vi "OOB Checker.vi"(8 "Deform Array":dbl[](array[numeric])=[1.0, 1.0, 1.0, 0.0, 0.0, 0.0, 0.0, 0.0, 0.0], 9 "Eye Model Cluster":T2={"X Grid"=[], "Y Grid"=[], "Za_true Surf"=[], "Iris Center"=[], "Zp_true Surf"=[], "Pinv"=[[1.0, 0.0], [0.0, 1.0]], "za_true"=5.0, "za_work"=1.0, "zp_work"=-1.0, "zp_true"=-5.0}, 11 "Check Pt":dbl[](array[numeric])=[0.0, 0.0, 0.0]) -> (0 "Point Out of Bound":bool, 3 "Check Pt*":dbl[](array[numeric]))   [LabVIEW 2016]
uses:
  <vilib>/Analysis/Matrix/Datatypes/RealMatrix.ctl
  <vilib>/Analysis/baseanly.llb/A x Vector.vi
  Subsystems/Global Variables.vi
  <vilib>/Analysis/baseanly.llb/Real Inverse Matrix.vi
  <vilib>/Analysis/7linalg.llb/Create Special Real Matrix.vi
  <vilib>/Analysis/NI_AALBase.lvlib
  <vilib>/Analysis/NI_AALPro.lvlib
  <vilib>/Analysis/NI_AALBLAS.lvlib
  <vilib>/Analysis/Matrix/NI_Matrix.lvlib
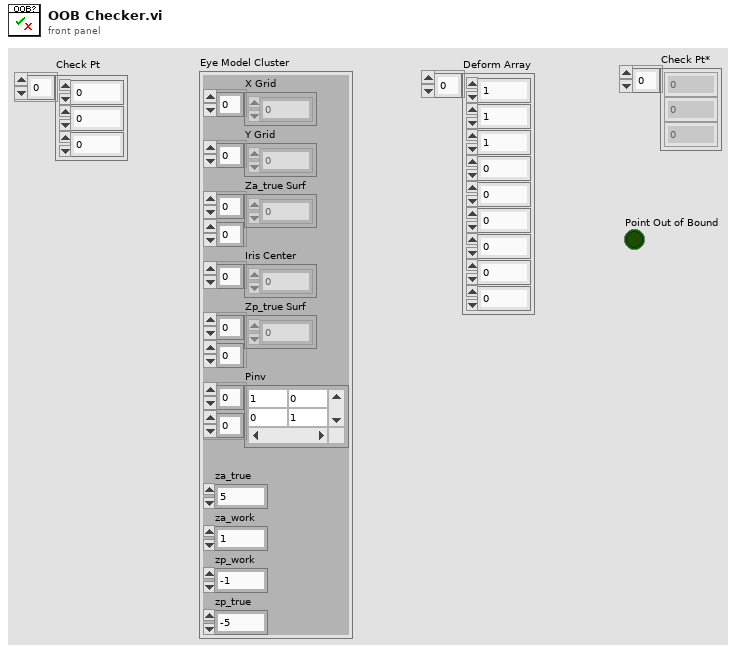
[diagram p1: front panel]
types:
  T1 = typedef "NI_Matrix.lvlib/RealMatrix.ctl" = dbl[][]
  T2 = cluster{"X Grid":dbl[], "Y Grid":dbl[], "Za_true Surf":dbl[][], "Iris Center":dbl[], "Zp_true Surf":dbl[][], "Pinv":T1, "za_true":dbl, "za_work":dbl, "zp_work":dbl, "zp_true":dbl}
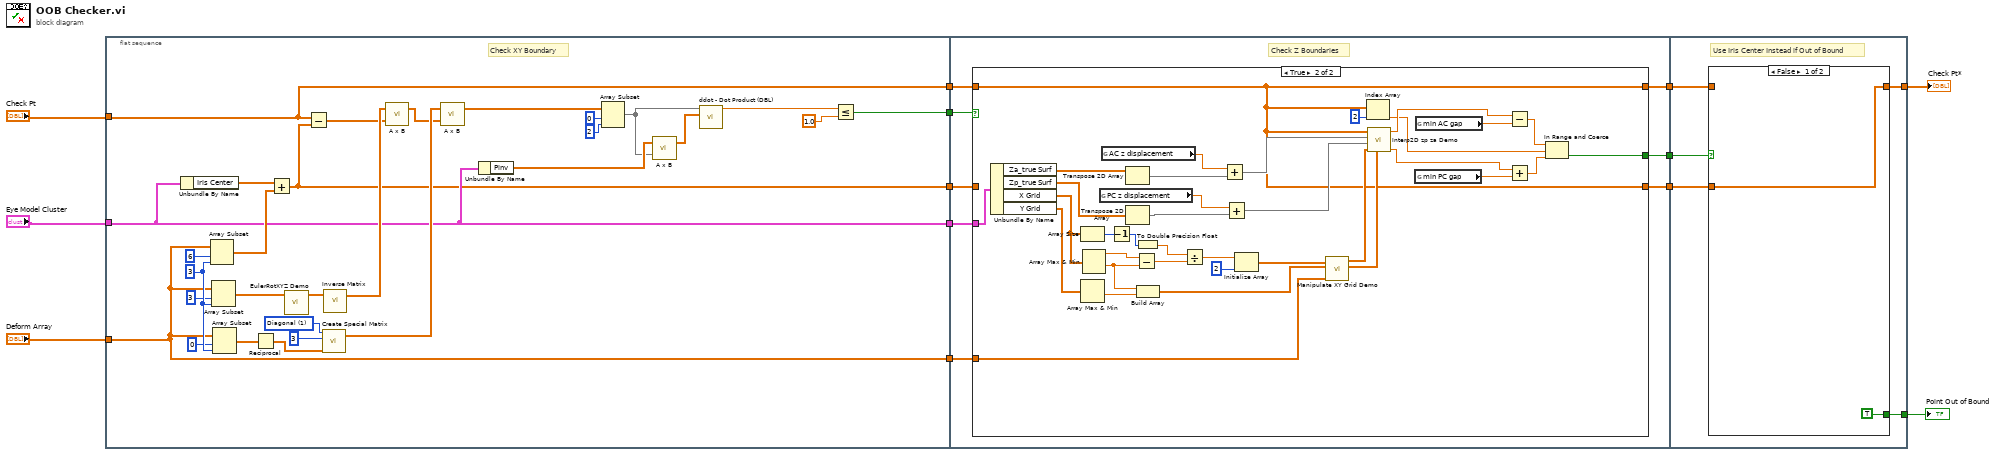
[diagram p0: block diagram]
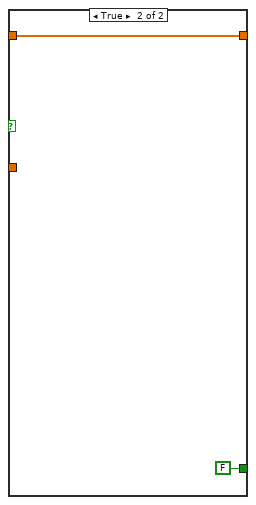
[diagram p3: hidden frame]
diagram:
  n1 = flat-sequence {
    tunnel: [w23] -> w13
    tunnel: [w15] -> w12
    tunnel: [w16] -> w11
    tunnel: [w17] -> w10
    tunnel: "Deform Array" -> [w17]
    tunnel: "Check Pt" -> [w15]
    tunnel: "Eye Model Cluster" -> [w16]
    tunnel: [w14] -> w4
    tunnel: w13 -> [w50]
    tunnel: w12 -> [w48]
    tunnel: w11 -> [w49]
    tunnel: w10 -> [w47]
    tunnel: [w46] -> w9
    tunnel: [w45] -> w8
    tunnel: w4 -> [w44]
    tunnel: [w43] -> w2
    tunnel: w9 -> [w93]
    tunnel: [w92] -> w3
    tunnel: w8 -> [w90]
    tunnel: [w91] -> w1
    tunnel: w2 -> [w89]
    frame #0 {
      w31 = 1 items=["Identity", "Diagonal", "Toeplitz", "Vandermonde", "Companion", "Hankel", "Hadamard", "Wilkinson", "Hilbert", "Inverse Hilbert", "Rosser", "Pascal"] ("matrix type")
      w41 = 3 ("length")
      # "Check XY Boundary"
      n2 = Unbundle By Name(w16) -> ("Iris Center"=w28:dbl[])
      n3 = Array Subset(array=w17, index=6 ("length"), length=w41) -> (w27:dbl[])
      n4 = Array Subset(array=w17, index=3, length=w41) -> (w38:dbl[])
      n5 = Array Subset(array=w17, index=0, length=w41) -> (w34:dbl[])
      n6 = Reciprocal(x=w34) -> (1/x=w33:dbl[])
      n7 = Add(x=w28, y=w27) -> (x+y=w14:dbl[])
      n8 = call "EulerRotXYZ Demo.vi"("Euler Angle (XYZ)"=w38) -> ("Rotation Mtx"=w37:T1)  [unwired: 10 in]
      n9 = Subtract(x=w15, y=w14) -> (x-y=w35:dbl[])
      n10 = call-poly <vilib>:"Create Special Matrix.vi"("matrix type"=w31, "matrix size"=3, "Input Vector1"=w33) -> ("Special Matrix"=w30:T1)  [unwired: 2 in, 1 out]
      n11 = call-poly <vilib>:"Inverse Matrix.vi"("Input Matrix"=w37) -> ("Inverse Matrix"=w36:T1)  [unwired: 1 in, 1 out]
      n12 = call-poly <vilib>:"A x B.vi"("Vector"=w35, "A"=w36) -> ("A x Vector"=w29:dbl[])  [unwired: 1 out]
      n13 = call-poly <vilib>:"A x B.vi"("Vector"=w29, "A"=w30) -> ("A x Vector"=w22:dbl[])  [unwired: 1 out]
      n14 = Unbundle By Name(w16) -> ("Pinv"=w19:T1)
      n15 = Array Subset(array=w22, index=0, length=2) -> (w18:dbl[])
      n16 = call-poly <vilib>:"A x B.vi"("Vector"=w18, "A"=w19) -> ("A x Vector"=w26:dbl[])  [unwired: 1 out]
      n17 = call <vilib>:"ddot - Dot Product (DBL).vi"("y"=w26, "x"=w18) -> ("ddot"=w25:dbl)  [unwired: 8 in, 1 out]
      n18 = Less Or Equal?(x=w25, y=1.0) -> (x <= y?=w23:bool)
    }
    frame #1 {
      # "Check Z Boundaries"
      n19 = case shown="True" w50 {
        selector: w50 -> [w53 _]
        tunnel: w49 -> [_ w81]
        tunnel: w48 -> [w51 w54]
        tunnel: w47 -> [_ w74]
        tunnel: [w53 w55] -> w46
        tunnel: [w52 w54] -> w45
        tunnel: w44 -> [w52 _]
        tunnel: [w51 w54] -> w43
        frame False {
        }
        frame True {
          n20 = Unbundle By Name(w81) -> ("Za_true Surf"=w67:dbl[][], "Zp_true Surf"=w65:dbl[][], "X Grid"=w80:dbl[], "Y Grid"=w79:dbl[])
          n21 = Array Size(array=w80) -> (size(s)=w82:i32)
          n22 = Array Max & Min(array=w79) -> (min value=w85:dbl)  [unwired: 3 out]
          n23 = Array Max & Min(array=w80) -> (max value=w84:dbl, min value=w83:dbl)  [unwired: 2 out]
          n24 = global read "Global Variables.vi" "PC z displacement"() -> (w72:dbl)
          n25 = global read "Global Variables.vi" "AC z displacement"() -> (w73:dbl)
          n26 = Decrement(x=w82) -> (x-1=w87:i32)
          n27 = Transpose 2D Array(2D array=w67) -> (transposed array=w66:dbl[][])
          n28 = Transpose 2D Array(2D array=w65) -> (transposed array=w64:dbl[][])
          n29 = Subtract(x=w84, y=w83) -> (x-y=w88:dbl)
          n30 = To Double Precision Float(number=w87) -> (double precision float=w86:dbl)
          n31 = Build Array(w83, w85) -> (w75:dbl[])
          n32 = Divide(x=w86, y=w88) -> (x/y=w77:dbl)
          n33 = Add(x=w73, y=w66) -> (x+y=w71:dbl[][])
          n34 = Add(x=w72, y=w64) -> (x+y=w70:dbl[][])
          n35 = Initialize Array(w77, 2 ("dimension size")) -> (w76:dbl[])
          n36 = call "Manipulate XY Grid Demo.vi"("Deform Array"=w74, "XY Grid min In"=w75, "XY Quant. Fact. In"=w76) -> ("XY Grid min Out"=w68:dbl[], "XY Quant. Fact. Out"=w69:dbl[])  [unwired: 7 in]
          n37 = Index Array(array=w54, index=2) -> (element=w56:dbl)
          n38 = call "Interp2D zp za Demo.vi"("XY Grid min"=w68, "XY Quantization Factor"=w69, "Zp array"=w70, "Za array"=w71, "Tip Position"=w54) -> ("zp"=w59:dbl, "za"=w60:dbl)  [unwired: 5 in]
          n39 = global read "Global Variables.vi" "min PC gap"() -> (w61:dbl)
          n40 = global read "Global Variables.vi" "min AC gap"() -> (w62:dbl)
          n41 = Subtract(x=w60, y=w62) -> (x-y=w58:dbl)
          n42 = Add(x=w59, y=w61) -> (x+y=w57:dbl)
          n43 = In Range and Coerce(upper limit=w58, x=w56, lower limit=w57) -> (In Range?=w55:bool)  [unwired: 1 out]
        }
      }
    }
    frame #2 {
      # "Use Iris Center Instead if Out of Bound"
      n44 = case shown="False" w93 {
        tunnel: [TRUE FALSE] -> w92
        tunnel: w90 -> [w94 _]
        tunnel: [w94 w96] -> w91
        tunnel: w89 -> [_ w96]
        frame False {
        }
        frame True {
        }
      }
    }
  }
  "Point Out of Bound" <- w3
  "Check Pt*" <- w1
